vi "SNF_Digital_Updated20181221.vi"() -> ()   [LabVIEW 2017]
uses:
  Users/Darcy/Documents/LabVIEW Data/MathScriptVIs/MCStatic_38597428832_1f828b6118eee4aae6c26f87bca7dc42.vi
  <instcachedir>/0/MCStatic_38597428832_1f828b6118eee4aae6c26f87bca7dc42_41DD7FBF8E354214ACC4B2D677C2F60C.lvgen/MCStatic_38597428832_1f828b6118eee4aae6c26f87bca7dc42_41DD7FBF8E354214ACC4B2D677C2F60C_000.vi
  <vilib>/imath/engines/lvmath2/RunTimeEngine/IndexRead/NIMS V(S).vi
  <instcachedir>/0/NIMS V(S)_0488751826AF41519A22953C041130DC.lvgen/NIMS V(S)_0488751826AF41519A22953C041130DC_000.vi
  <vilib>/imathl/engines/lvmath/Functions/Error Handling/Create Error.vi
  <vilib>/imath/engines/lvmath2/RunTimeEngine/NodeEndStatement/NIMS_NodeEndStatement_Output.vi
  <instcachedir>/0/NIMS_NodeEndStatement_Output_53EC0D466D134D7ABD903AC30B43404B.lvgen/NIMS_NodeEndStatement_Output_53EC0D466D134D7ABD903AC30B43404B_001.vi
  <instcachedir>/0/NIMS_NodeEndStatement_Output_53EC0D466D134D7ABD903AC30B43404B.lvgen/NIMS_NodeEndStatement_Output_53EC0D466D134D7ABD903AC30B43404B_005.vi
  <vilib>/imath/engines/lvmath2/RunTimeEngine/ErrorHandling/NIMS_Finalize Error.vi
  <vilib>/Utility/file.llb/Read Delimited Spreadsheet (DBL).vi
  Users/Darcy/Documents/LabVIEW Data/reactor_power.m
  Users/Darcy/Documents/LabVIEW Data/long_term_power.m
  Users/Darcy/Documents/LabVIEW Data/power_function.m
  Users/Darcy/Documents/LabVIEW Data/short_term_power.m
panel:
  out "Control Rod Out":dbl(graph)
  out "Rod In:":dbl(slide) caption="Power Output [W]"
  out "Rod Out:":dbl(slide) caption="Power Output [W]" scale=0.0..1.0
  out "Power [W]":dbl(slide) caption="Power Output [W]" scale=0.0..10000.0
  out "SNF Desired Power":dbl(graph)
  in  "Fine Gain Value":dbl(slide)=0.0009918367346938776 scale=0.0001..0.002
  out "T_Coolant (C)":dbl
  out "SNFDesiredPower":dbl=50.0
  in  "Input Steady State:":dbl=0.644 format="%#_13g"
  in  "Input Amplitude:":dbl=0.001
  in  "Initial Power:":dbl=8000.0 format="%#_13g"
  in  "Maximum Power:":dbl=10000.0
  in  "Minimum Power:":dbl=1.0
  out "T_Fuel (C)":dbl
  out "Coolant Temp":dbl(slide) scale=0.0..200.0
  out "Fuel Temp":dbl(slide) scale=0.0..200.0
  in  "Input Length":dbl
  out "Iterations":dbl
  in  "?":bool
  in  "?":bool
  out "Array":dbl[](array[numeric])
  in  "INPUT/MANUAL":bool=TRUE
  in  "Load Power Profile":bool
  in  "Dyn. Control Rod Profile File":path
  in  "?":bool
  in  "Equilibrium T_Coolant\nFHR: 100":dbl=100.0
  in  "Equilibrium T_Fuel\nFHR: 100":dbl=100.0
  in  "Coolant Feedback Coef\nFHR: -2.1":dbl=-2.1
  in  "Fuel Feedback Coef\nFHR: -6.7":dbl=-6.7
  in  "CRW Coef":dbl=0.005
  in  "CRW Constant":dbl=0.999
  in  "beta\nFHR: 0.0065":dbl=0.0065
  in  "Lambda\nFHR: 5.02e-4":dbl=0.000502
  in  "lambda\nFHR: 0.0785":dbl=0.0785
  out "Net Reactivity":dbl
  out "Rod Reactivity":dbl
  out "Net Rod Out":dbl
  in  "SCRAM":bool
  out "Resolution":dbl=0.05
  out "Control Rod Out":dbl=0.644
  in  "STOP TOGGLE":bool
  # "Neutronics"
  # "Control Rod Worth (CRW)"
  # "Fine"
  # "Coarse"
  # "Temperature Feedback"
  # "Manual"
  # "Input"
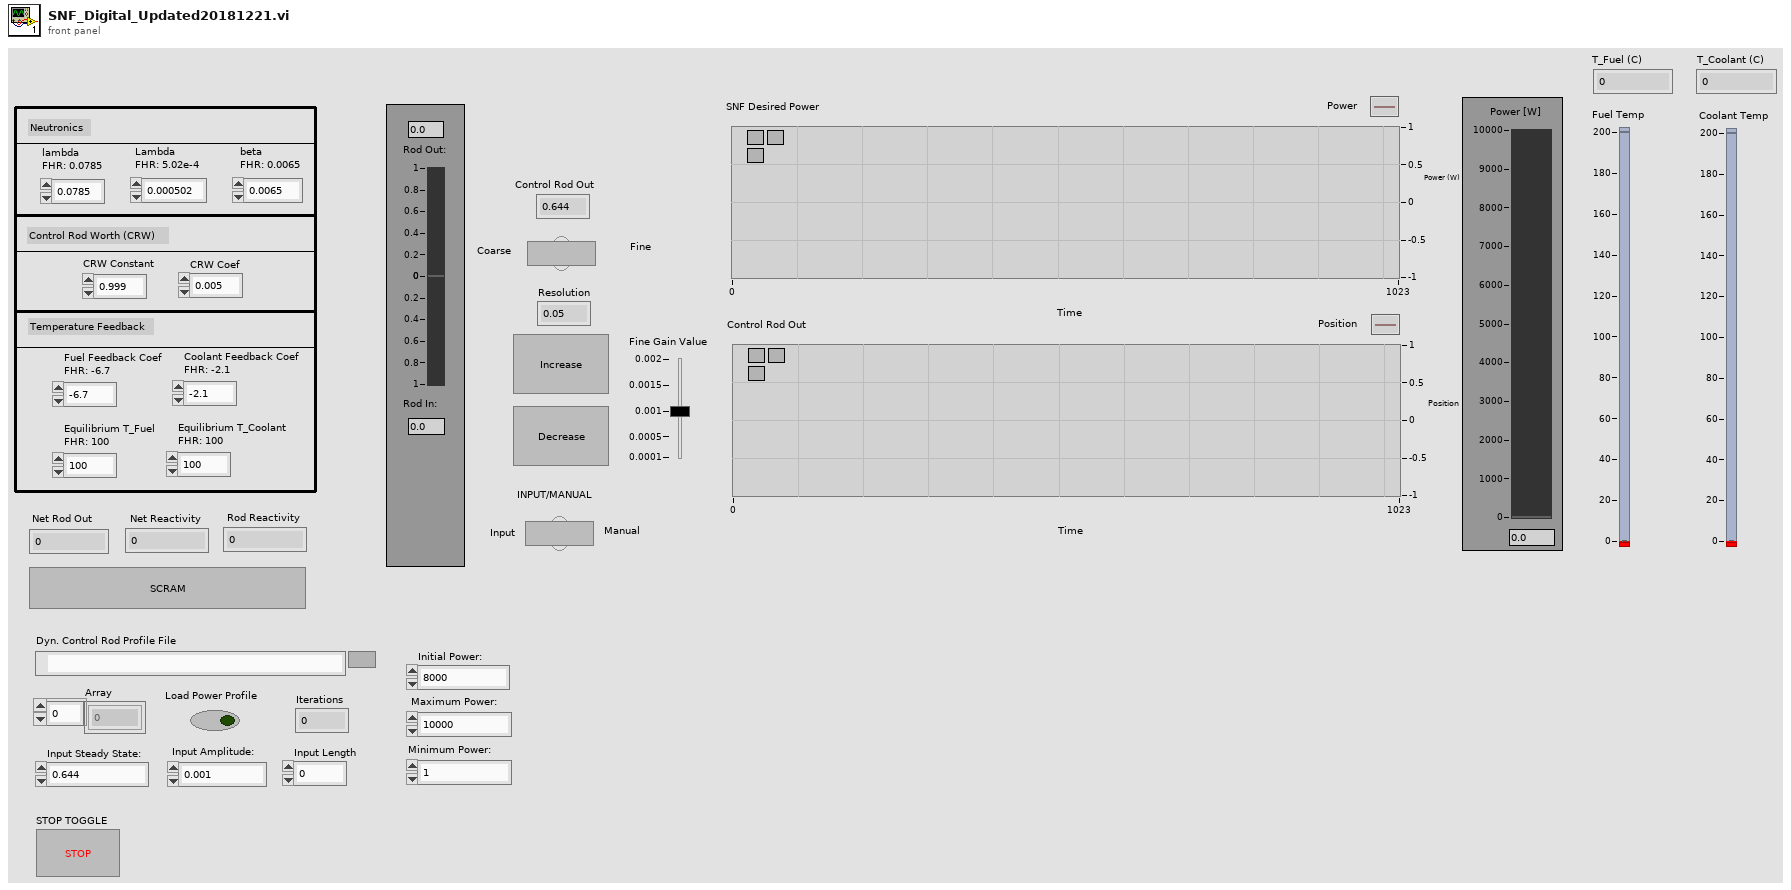
[diagram p1: front panel]
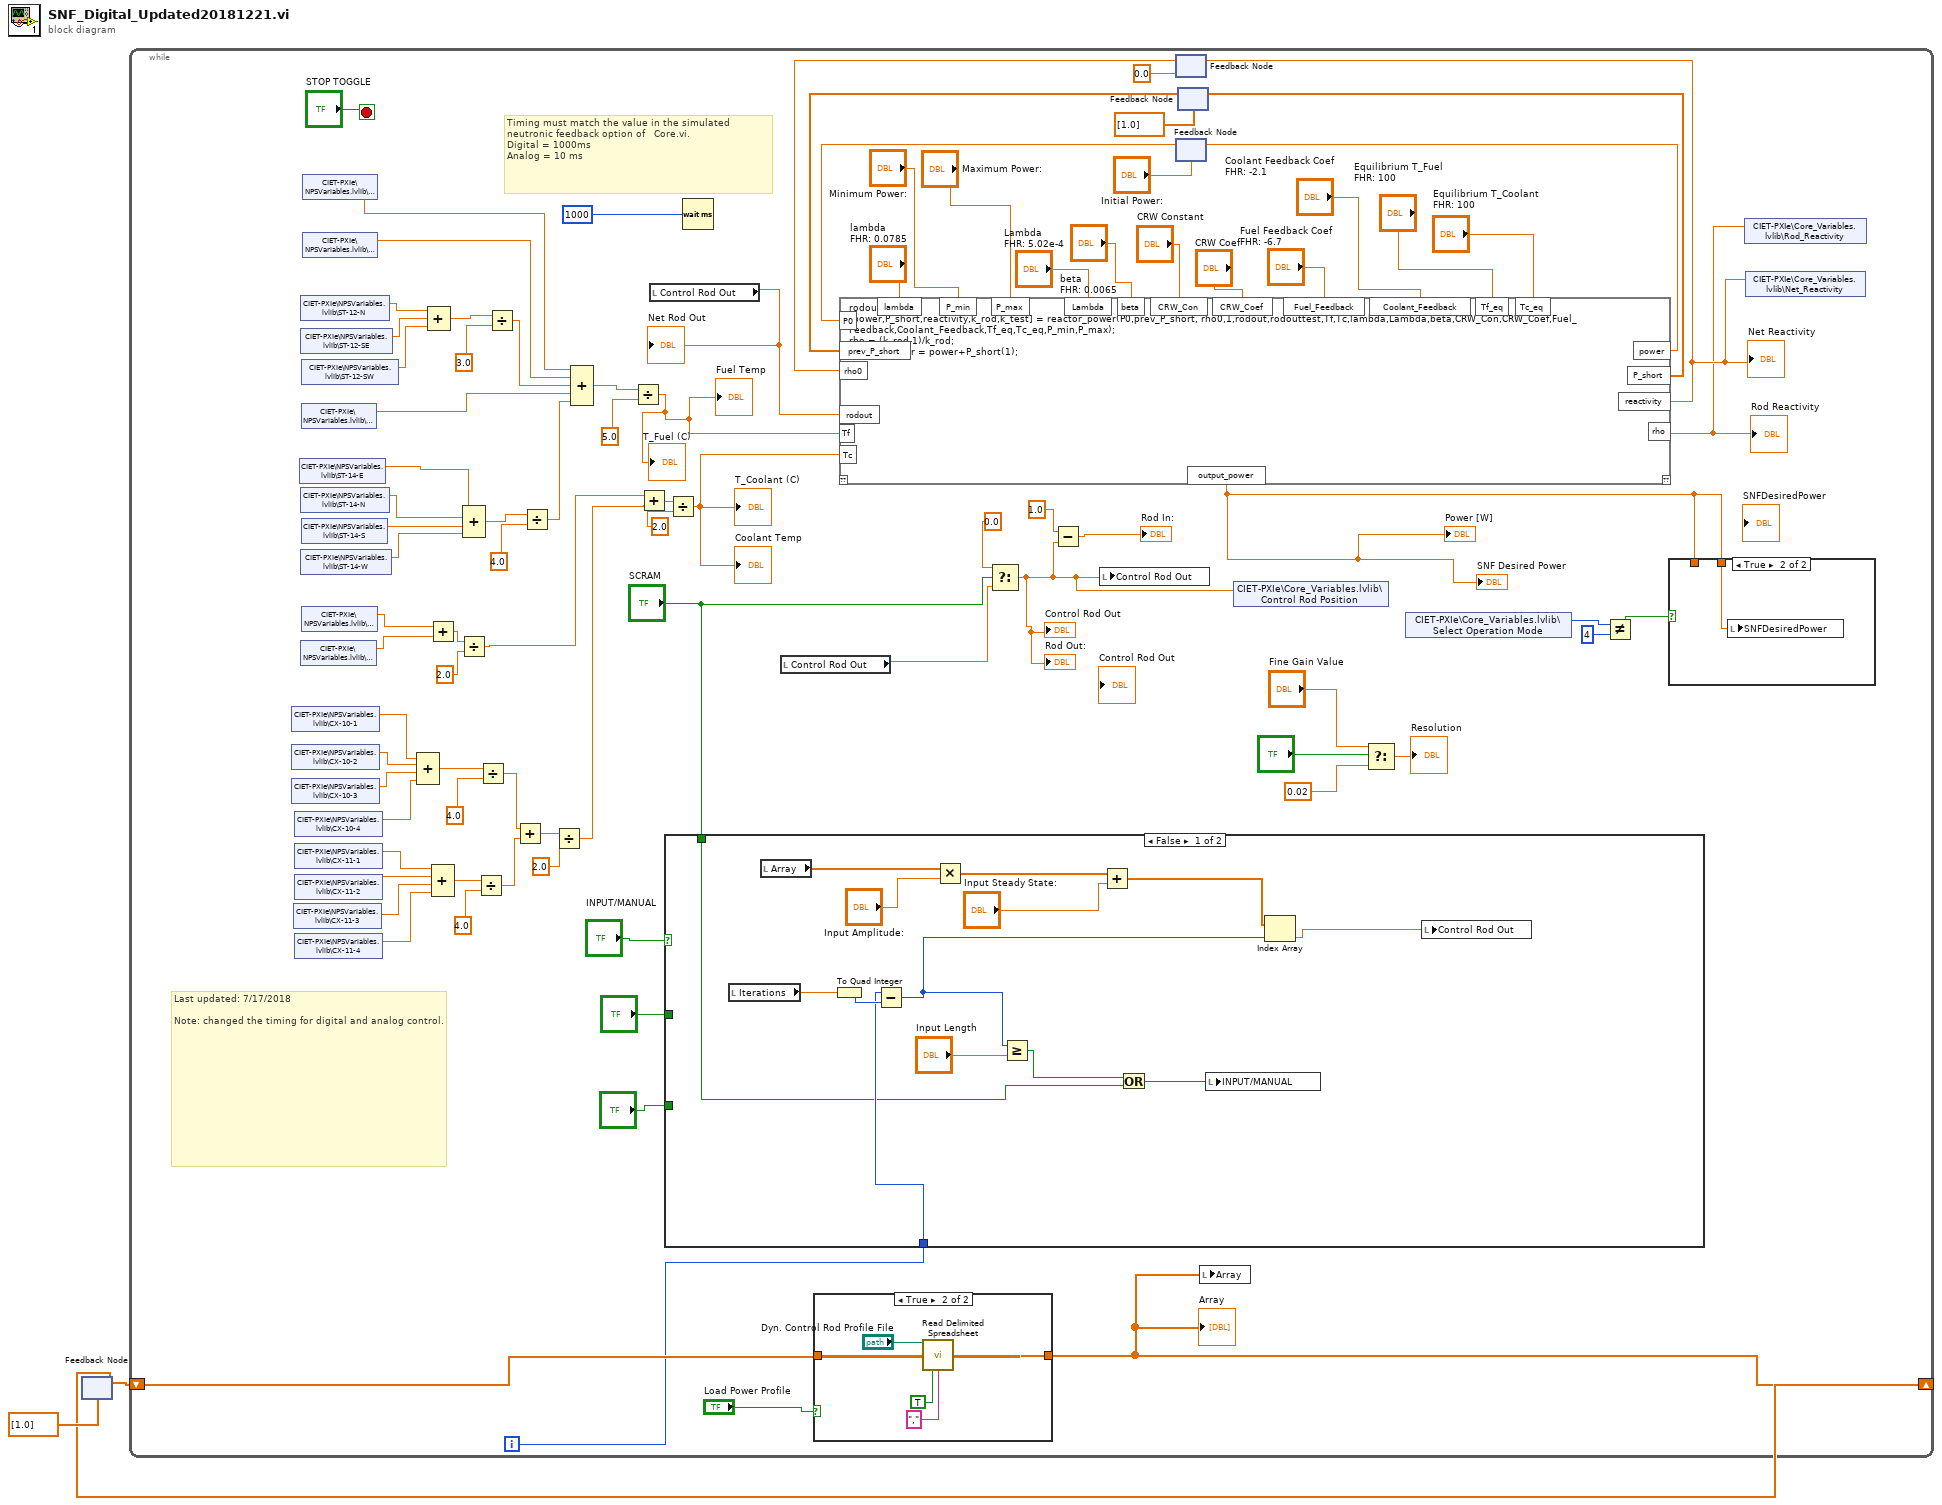
[diagram p0: block diagram]
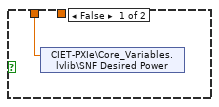
[diagram p2: hidden frame]
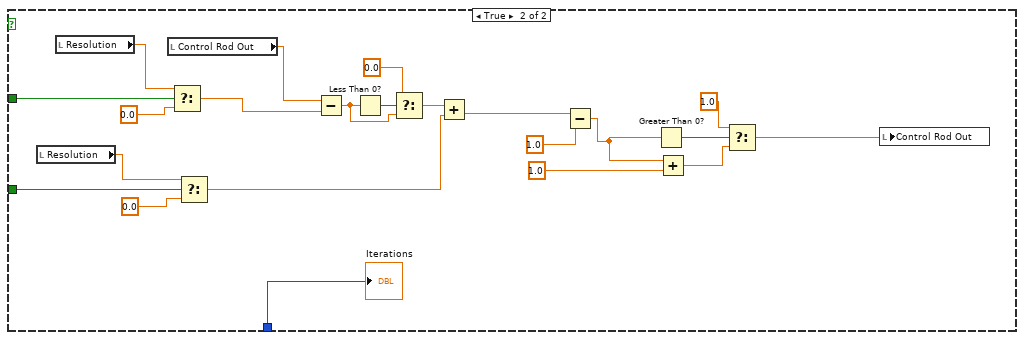
[diagram p3: hidden frame]
diagram:
  n1 = feedback #1(dbl[] [1.0] ("P_short")) -> (w3:dbl[])
  n2 = while {
    shift-right: [w66] -> w1
    shift-left: w3 -> [w67]
    i -> [w61]
    stop <- "STOP TOGGLE" stop-if-true
    # "Last updated: 7/17/2018\n\nNote: changed the timing for digital and analog control."
    # "Timing must match the value in the simulated neutronic feedback option of   Core.vi. \nDigital = 1000ms \nAnalog = 10 ms"
    n3 = shared-variable "CIET-PXIe\\NPSVariables.lvlib\\CX-10-1"() -> (w26:sgl)  [unwired: 1 in, 1 out]
    n4 = shared-variable "CIET-PXIe\\NPSVariables.lvlib\\CX-10-2"() -> (w25:sgl)  [unwired: 1 in, 1 out]
    n5 = shared-variable "CIET-PXIe\\NPSVariables.lvlib\\CX-10-3"() -> (w24:sgl)  [unwired: 1 in, 1 out]
    n6 = shared-variable "CIET-PXIe\\NPSVariables.lvlib\\CX-11-3"() -> (w20:sgl)  [unwired: 1 in, 1 out]
    n7 = shared-variable "CIET-PXIe\\NPSVariables.lvlib\\CX-10-4"() -> (w23:sgl)  [unwired: 1 in, 1 out]
    n8 = shared-variable "CIET-PXIe\\NPSVariables.lvlib\\CX-11-1"() -> (w22:sgl)  [unwired: 1 in, 1 out]
    n9 = shared-variable "CIET-PXIe\\NPSVariables.lvlib\\CX-11-2"() -> (w21:sgl)  [unwired: 1 in, 1 out]
    n10 = shared-variable "CIET-PXIe\\NPSVariables.lvlib\\CX-11-4"() -> (w19:sgl)  [unwired: 1 in, 1 out]
    n11 = shared-variable "CIET-PXIe\\NPSVariables.lvlib\\ST-14-E"() -> (w41:sgl)  [unwired: 1 in, 1 out]
    n12 = shared-variable "CIET-PXIe\\NPSVariables.lvlib\\ST-12-N"() -> (w48:sgl)  [unwired: 1 in, 1 out]
    n13 = shared-variable "CIET-PXIe\\NPSVariables.lvlib\\ST-12-SE"() -> (w47:sgl)  [unwired: 1 in, 1 out]
    n14 = shared-variable "CIET-PXIe\\NPSVariables.lvlib\\ST-14-N"() -> (w40:sgl)  [unwired: 1 in, 1 out]
    n15 = shared-variable "CIET-PXIe\\NPSVariables.lvlib\\ST-14-W"() -> (w38:sgl)  [unwired: 1 in, 1 out]
    n16 = shared-variable "CIET-PXIe\\NPSVariables.lvlib\\BT-12"() -> (w55:sgl)  [unwired: 1 in, 1 out]
    n17 = shared-variable "CIET-PXIe\\NPSVariables.lvlib\\ST-12-SW"() -> (w46:sgl)  [unwired: 1 in, 1 out]
    n18 = shared-variable "CIET-PXIe\\NPSVariables.lvlib\\ST-13"() -> (w44:sgl)  [unwired: 1 in, 1 out]
    n19 = shared-variable "CIET-PXIe\\NPSVariables.lvlib\\ST-14-S"() -> (w39:sgl)  [unwired: 1 in, 1 out]
    n20 = shared-variable "CIET-PXIe\\NPSVariables.lvlib\\BT-11"() -> (w56:sgl)  [unwired: 1 in, 1 out]
    n21 = shared-variable "CIET-PXIe\\NPSVariables.lvlib\\ST-10"() -> (w54:sgl)  [unwired: 1 in, 1 out]
    n22 = shared-variable "CIET-PXIe\\NPSVariables.lvlib\\ST-11"() -> (w53:sgl)  [unwired: 1 in, 1 out]
    n23 = Compound Arithmetic op=ADD(w26, w25, w24, w23) -> (w32:sgl)
    n24 = Compound Arithmetic op=ADD(w48, w47, w46) -> (w50:sgl)
    n25 = Add(x=w56, y=w55) -> (x+y=w58:sgl)
    n26 = Compound Arithmetic op=ADD(w22, w21, w20, w19) -> (w30:sgl)
    n27 = Divide(x=w58, y=2.0) -> (x/y=w35:dbl)
    n28 = Compound Arithmetic op=ADD(w41, w40, w39, w38) -> (w43:sgl)
    n29 = Divide(x=w30, y=4.0) -> (x/y=w27:dbl)
    n30 = Divide(x=w32, y=4.0) -> (x/y=w28:dbl)
    n31 = Divide(x=w50, y=3.0) -> (x/y=w45:dbl)
    n32 = Add(x=w28, y=w27) -> (x+y=w60:dbl)
    n33 = Divide(x=w43, y=4.0) -> (x/y=w37:dbl)
    n34 = Divide(x=w60, y=2.0) -> (x/y=w34:dbl)
    n35 = Compound Arithmetic op=ADD(w54, w53, w45, w44, w37) -> (w52:dbl)
    n36 = Divide(x=w52, y=5.0) -> (x/y=w18:dbl)
    "Fuel Temp" <- w18
    "T_Fuel (C)" <- w18
    n37 = Add(x=w35, y=w34) -> (x+y=w33:dbl)
    n38 = local read "Control Rod Out"() -> (w69:dbl)
    "Net Rod Out" <- w69
    n39 = case shown="False" "INPUT/MANUAL" {
      tunnel: "?" -> [_ w112]
      tunnel: "?" -> [_ w111]
      tunnel: w61 -> [w104 w110]
      tunnel: "SCRAM" -> [w102 _]
      frame False {
        n40 = local read "Iterations"() -> (w106:dbl)
        n41 = local read "Array"() -> (w99:dbl[])
        n42 = To Quad Integer(1:w106) -> (0:w105:i64)
        n43 = Subtract(x=w104, y=w105) -> (x-y=w107:i64)
        n44 = Multiply(x=w99, y="Input Amplitude:") -> (x*y=w97:dbl[])
        n45 = Greater Or Equal?(x=w107, y="Input Length") -> (x >= y?=w103:bool)
        n46 = Add(x=w97, y="Input Steady State:") -> (x+y=w95:dbl[])
        n47 = Or(x=w103, y=w102) -> (x .or. y?=w101:bool)
        n48 = local write "INPUT/MANUAL"(w101) -> ()
        n49 = Index Array(array=w95, index=w107) -> (element=w100:dbl)
        n50 = local write "Control Rod Out"(w100) -> ()
      }
      frame True {
        n51 = local read "Resolution"() -> (w128:dbl)
        n52 = local read "Resolution"() -> (w130:dbl)
        n53 = local read "Control Rod Out"() -> (w126:dbl)
        n54 = Select(t=w130, s=w112, f=0.0) -> (s? t:f=w125:dbl)
        n55 = Select(t=w128, s=w111, f=0.0) -> (s? t:f=w113:dbl)
        n56 = Subtract(x=w126, y=w125) -> (x-y=w123:dbl)
        n57 = Less Than 0?(x=w123) -> (x < 0?=w124:bool)
        n58 = Select(t=0.0, s=w124, f=w123) -> (s? t:f=w121:dbl)
        n59 = Add(x=w121, y=w113) -> (x+y=w120:dbl)
        n60 = Subtract(x=w120, y=1.0) -> (x-y=w116:dbl)
        n61 = Greater Than 0?(x=w116) -> (x > 0?=w118:bool)
        n62 = Add(x=w116, y=1.0) -> (x+y=w115:dbl)
        n63 = Select(t=1.0, s=w118, f=w115) -> (s? t:f=w109:dbl)
        n64 = local write "Control Rod Out"(w109) -> ()
        "Iterations" <- w110
      }
    }
    n65 = Divide(x=w33, y=2.0) -> (x/y=w8:dbl)
    "Coolant Temp" <- w8
    "T_Coolant (C)" <- w8
    n66 = Wait (ms)(milliseconds to wait=u32 1000) -> ()  [unwired: 1 out]
    n67 = local read "Control Rod Out"() -> (w62:dbl)
    n68 = case shown="True" "Load Power Profile" {
      tunnel: [w131 w132] -> w66
      tunnel: w67 -> [w131 _]
      frame False {
      }
      frame True {
        n69 = call-poly <vilib>:"Read Delimited Spreadsheet.vi"("file path (dialog if empty)"="Dyn. Control Rod Profile File", "transpose? (F)"=TRUE, "delimiter (\\t)"="," ("delimiter (\\t)")) -> ("first row"=w132:dbl[])  [unwired: 7 in, 5 out]
      }
    }
    "Array" <- w66
    n70 = Select(t=0.0, s="SCRAM", f=w62) -> (s? t:f=w4:dbl)
    "Rod Out:" <- w4
    "Control Rod Out" <- w4
    n71 = Subtract(x=1.0, y=w4) -> (x-y=→"Rod In:":dbl)
    n72 = local write "Control Rod Out"(w4) -> ()
    n73 = feedback #2(0.0 ("reactivity")) -> (w85:dbl)
    n74 = feedback #3("Initial Power:") -> (w88:dbl)
    n75 = feedback #4(dbl[] [1.0] ("P_short")) -> (w86:dbl[])
    n76 = mathscript code="rodouttest = 0;\n[power,P_short,reactivity,k_rod,k_test] = reactor_power(P0,prev_P_short, rho0,1,rodout,rodouttest,Tf,Tc,lambda,Lambda,beta,CRW_Con,CRW_Coef,Fuel_Feedback,Coolant_Feedback,Tf_eq,Tc_eq,P_min,P_max);\nrho = (k_rod-1)/k_rod;\noutput_power = power+P_short(1);"("rodout"=w69, "P0"=w88, "prev_P_short"=w86, "rho0"=w85, "Tf"=w18, "Tc"=w8, "lambda"="lambda\nFHR: 0.0785", "Lambda"="Lambda\nFHR: 5.02e-4", "beta"="beta\nFHR: 0.0065", "CRW_Con"="CRW Constant", "CRW_Coef"="CRW Coef", "Fuel_Feedback"="Fuel Feedback Coef\nFHR: -6.7", "Coolant_Feedback"="Coolant Feedback Coef\nFHR: -2.1", "Tf_eq"="Equilibrium T_Fuel\nFHR: 100", "Tc_eq"="Equilibrium T_Coolant\nFHR: 100", "P_max"="Maximum Power:", "P_min"="Minimum Power:") -> ("power"=w89:dbl, "P_short"=w87:dbl[], "reactivity"=w14:dbl, "output_power"=w6:dbl, "rho"=w13:dbl)  [unwired: 1 in, 1 out]
    "Rod Reactivity" <- w13
    "Net Reactivity" <- w14
    "SNF Desired Power" <- w6
    "Power [W]" <- w6
    n77 = feedback-in #2(w14) -> ()
    n78 = feedback-in #3(w89) -> ()
    n79 = feedback-in #4(w87) -> ()
    n80 = local write "Array"(w66) -> ()
    n81 = shared-variable "CIET-PXIe\\Core_Variables.lvlib\\Control Rod Position"(w4) -> ()  [unwired: 1 in, 1 out]
    n82 = Select(t="Fine Gain Value", s="?", f=0.02) -> (s? t:f=→"Resolution":dbl)
    n83 = shared-variable "CIET-PXIe\\Core_Variables.lvlib\\Select Operation Mode"() -> (w10:u16)  [unwired: 1 in, 1 out]
    n84 = Not Equal?(x=w10, y=u16 4) -> (x != y?=w9:bool)
    n85 = case shown="True" w9 {
      tunnel: w6 -> [w93 _]
      tunnel: w6 -> [_ w94]
      frame False {
        n86 = shared-variable "CIET-PXIe\\Core_Variables.lvlib\\SNF Desired Power"(w93) -> ()  [unwired: 1 in, 1 out]
      }
      frame True {
        n87 = local write "SNFDesiredPower"(w94) -> ()
      }
    }
    n88 = shared-variable "CIET-PXIe\\Core_Variables.lvlib\\Rod_Reactivity"(w13) -> ()  [unwired: 1 in, 1 out]
    n89 = shared-variable "CIET-PXIe\\Core_Variables.lvlib\\Net_Reactivity"(w14) -> ()  [unwired: 1 in, 1 out]
  }
  n90 = feedback-in #1(w1) -> ()
